vi "ref_STRING_offset.vi"(10 "ST_reference_info":T1, 11 "STRING_position":i16) -> (3 "reference_byte_array_offset":i32)   [LabVIEW 2020]
uses:
  ST_reference_info.ctl
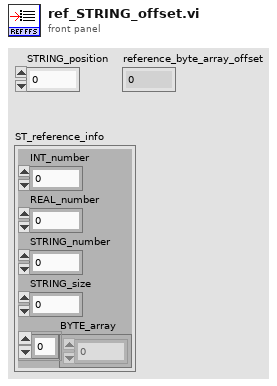
[diagram p1: front panel]
types:
  T1 = typedef "ST_reference_info.ctl" = cluster{"INT_number":i32, "REAL_number":i32, "STRING_number":i32, "STRING_size":i32, "BYTE_array":u8[]}
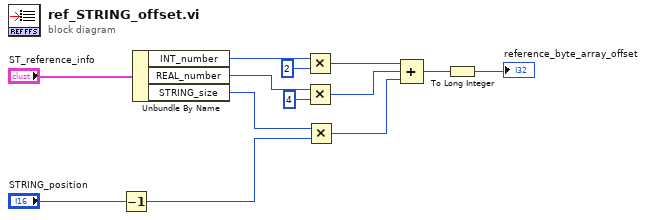
[diagram p0: block diagram]
diagram:
  n1 = Decrement(x="STRING_position") -> (x-1=w1:i16)
  n2 = Unbundle By Name("ST_reference_info") -> ("INT_number"=w11:i32, "REAL_number"=w9:i32, "STRING_size"=w7:i32)
  n3 = Multiply(x=w11, y=2) -> (x*y=w6:i32)
  n4 = Multiply(x=w9, y=4) -> (x*y=w5:i32)
  n5 = Multiply(x=w7, y=w1) -> (x*y=w4:i32)
  n6 = Compound Arithmetic op=ADD(w6, w5, w4) -> (w3:i32)
  n7 = To Long Integer(number=w3) -> (32bit integer=→"reference_byte_array_offset":i32)
